vi "detrend.VI"(1 "数据序列":dbl[](array[numeric]) format="%.2f") -> (0 "处理后的数据序列":dbl[](graph))   [LabVIEW 2010]
uses:
  <vilib>/Analysis/NI_AALPro.lvlib
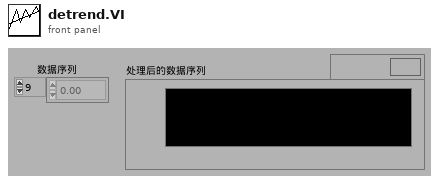
[diagram p1: front panel]
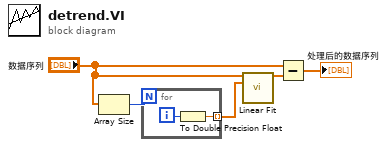
[diagram p0: block diagram]
diagram:
  n1 = Array Size(array="数据序列") -> (size(s)=w5:i32)
  n2 = for {
    N: w5 -> [_]
    tunnel: [w6] -> w1 mode=indexing
    i -> [w7]
    n3 = To Double Precision Float(number=w7) -> (double precision float=w6:dbl)
  }
  n4 = call <vilib>:"Linear Fit.vi"("Y"="数据序列", "X"=w1) -> ("Best Linear Fit"=w4:dbl[])  [unwired: 9 in, 4 out]
  n5 = Subtract(x="数据序列", y=w4) -> (x-y=→"处理后的数据序列":dbl[])
